vi "相连的移位寄存器.vi"() -> ()   [LabVIEW 2020]
doc: "本VI是为《我和LabVIEW》一书编写的示例。\n关于本书的介绍请参考网页：\nhttp://ruanqizhen.spaces.live.com/blog/cns!5852D4F797C53FB6!4310.entry"
panel:
  in  "数组":string[](array[string])
  out "输出整数":i32
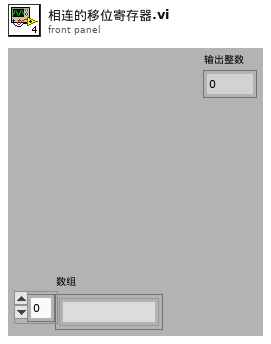
[diagram p1: front panel]
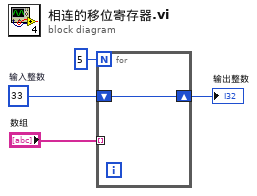
[diagram p0: block diagram]
diagram:
  w4 = 33  # 输入整数
  n1 = for {
    N: 5 -> [_]
    tunnel: "数组" -> [_] mode=indexing
    shift-right: [w5] -> w2
    shift-left: w4 -> [w5]
  }
  "输出整数" <- w2
